vi "ManualControlL0NoLoop.vi"() -> ()   [LabVIEW 2009]
uses:
  <vilib>/Utility/NIReport.llb/NI_report.lvclass
  <vilib>/Utility/NIReport.llb/HTML/NI_HTML.lvclass
panel:
  in  "Amp Scaler":dbl(slide)=1.110204081632653 scale=0.1..10.0
  in  "Voltage Input":dbl(slide)=0.21071428571428574 scale=0.05..0.8
  in  "Sum/Maj":bool=TRUE
  in  "Ib Clip select":i32(slide)=63 scale=0.0..63.0
  in  "Clipping Select":i32(slide)=1 scale=1.0..3.0
  in  "Attenuation Select":i32(slide) scale=0.0..15.0
  in  "Delay Enable":i32(slide) scale=0.0..31.0
  in  "Channel Enable":i32(slide) scale=0.0..6.0
  in  "Instrument VISA in":T1={"AWG VISA"="generadorpulsos", "Oscilloscope  VISA "="Oscilloscope", "Integration Board IP"="172.16.7.43", "connection ID"=refnum, "report out"=refnum, "report file path"=path "C:/Documents and Settings/CTA_LAB01/Desktop/L0_Asic/L0 Asic Test Data"}
  out "error out":errorcluster
  in  "error in (no error)":errorcluster
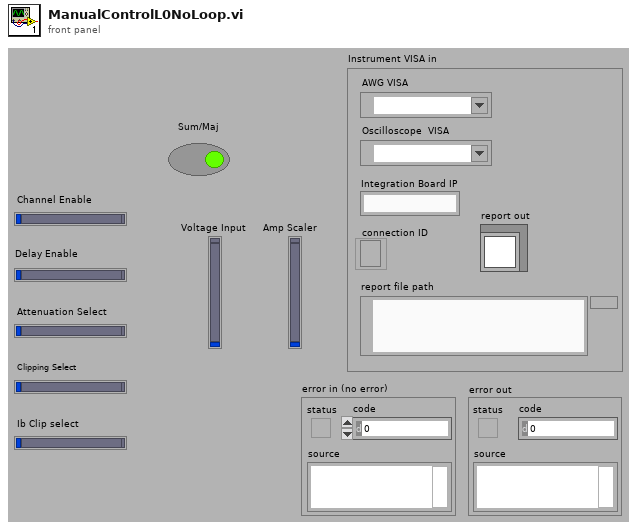
[diagram p1: front panel]
types:
  T1 = cluster{"AWG VISA":refnum<visa-resource-name>, "Oscilloscope  VISA ":refnum<visa-resource-name>, "Integration Board IP":string, "connection ID":refnum<k5>, "report out":refnum<class "NI_report.lvclass">, "report file path":path}
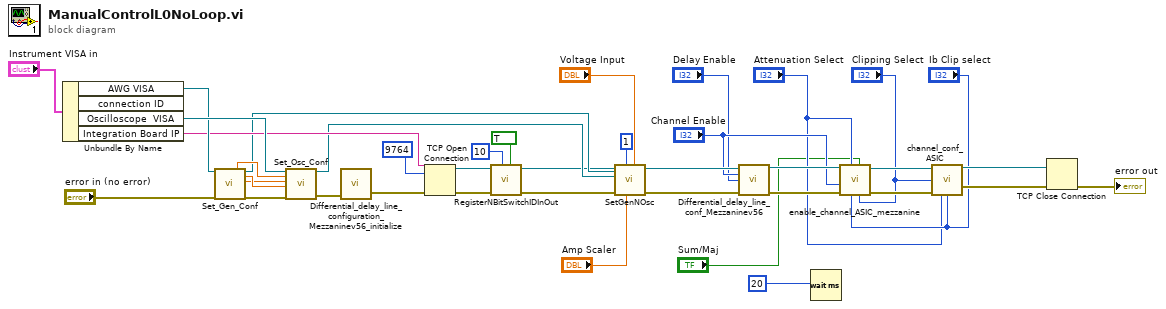
[diagram p0: block diagram]
diagram:
  n1 = Unbundle By Name("Instrument VISA in") -> ("AWG VISA"=w33:refnum<visa-resource-name>, "Oscilloscope  VISA"=w34:refnum<visa-resource-name>, "Integration Board IP"=w32:string)  [unwired: 1 out]
  n2 = call "Set_Gen_Conf.vi"("AWG VISA"=w33, "error in (no error)"="error in (no error)") -> ("Amplitude 1 OUT"=w30:dbl, "VISA resource name out"=w21:refnum<visa-resource-name>, "Pulse Width in seconds 1 OUT"=w29:dbl, "Trigger Level 1"=w28:dbl, "error out"=w36:errorcluster)  [unwired: 10 in, 3 out]
  n3 = call "Set_Osc_Conf.vi"("VISA resource name"=w34, "Amplitude IN"=w30, "Trigger Level IN"=w28, "Pulse Width in seconds IN"=w29, "error in (no error)"=w36) -> ("VISA resource name out"=w22:refnum<visa-resource-name>, "error out"=w27:errorcluster)  [unwired: 13 in]
  n4 = call "Differential_delay_line_configuration_Mezzaninev56_initialize.vi"("error in (no error)"=w27) -> ("error out 2"=w26:errorcluster)  [unwired: 1 in]
  n5 = TCP Open Connection(address=w32, remote port or service name=9764, error in (no error)=w26) -> (connection ID=w19:refnum<k5>, error out=w25:errorcluster)  [unwired: 2 in]
  n6 = call "RegisterNBitSwitchIDInOut.vi"("Switch Bit"=TRUE, "N Bit"=10, "error in (no error)"=w25, "connection ID"=w19) -> ("error out"=w20:errorcluster, "connection ID out"=w18:refnum<k5>)  [unwired: 5 in]
  n7 = call "SetGenNOsc.vi"("Input Voltage"="Voltage Input", "Amp Scaler"="Amp Scaler", "NChannels"=1, "error in (no error)"=w20, "VISA resource name"=w22, "AWG VISA"=w21) -> ("error out 2"=w4:errorcluster)  [unwired: 5 in]
  n8 = call "Differential_delay_line_conf_Mezzaninev56.vi"("connection ID"=w18, "channel"="Channel Enable", "Delay value"="Delay Enable", "error in (no error)"=w4) -> ("connection ID out"=w13:refnum<k5>, "error out 2"=w15:errorcluster)  [unwired: 4 in, 6 out]
  n9 = Wait (ms)(milliseconds to wait=20) -> ()  [unwired: 1 out]
  n10 = call "enable_channel_ASIC_mezzanine.vi"("Clip_sel_b"="Clipping Select", "maj/sum"="Sum/Maj", "Ib_clipVb"="Ib Clip select", "Att gain"="Attenuation Select", "error in"=w15, "Channel"="Channel Enable", "connection ID"=w13) -> ("error out"=w14:errorcluster, "connection ID out"=w12:refnum<k5>)  [unwired: 2 in, 1 out]
  n11 = call "channel_conf_ASIC.vi"("connection ID"=w12, "Clip_sel_b"="Clipping Select", "error out"=w14, "Att gain"="Attenuation Select", "Ib_ClipVb"="Ib Clip select") -> ("connection ID out"=w23:refnum<k5>, "error out 2"=w24:errorcluster)  [unwired: 6 in, 3 out]
  n12 = TCP Close Connection(connection ID=w23, error in (no error)=w24) -> (error out=→"error out":errorcluster)  [unwired: 1 in, 1 out]
